vi "GenPointAttay.vi"(8 "error in":errorcluster, 11 "Option":T1={"X個數"=20, "Y個數"=10, "起始X"=0.0, "起始Y"=0.0, "位移X"=20.0, "位移Y"=20.0, "抖動range"=0.0}) -> (0 "error out":errorcluster, 3 "Output Points":cluster{"X":dbl, "Y":dbl}[](array[cluster]))   [LabVIEW 2015]
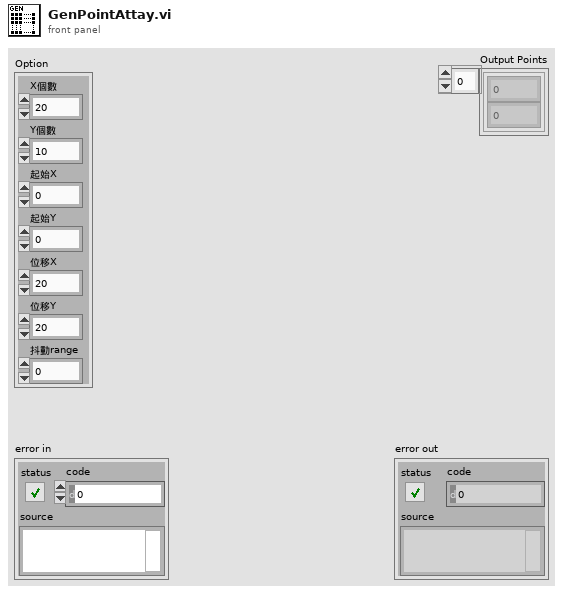
[diagram p1: front panel]
types:
  T1 = cluster{"X個數":i32, "Y個數":i32, "起始X":dbl, "起始Y":dbl, "位移X":dbl, "位移Y":dbl, "抖動range":dbl}
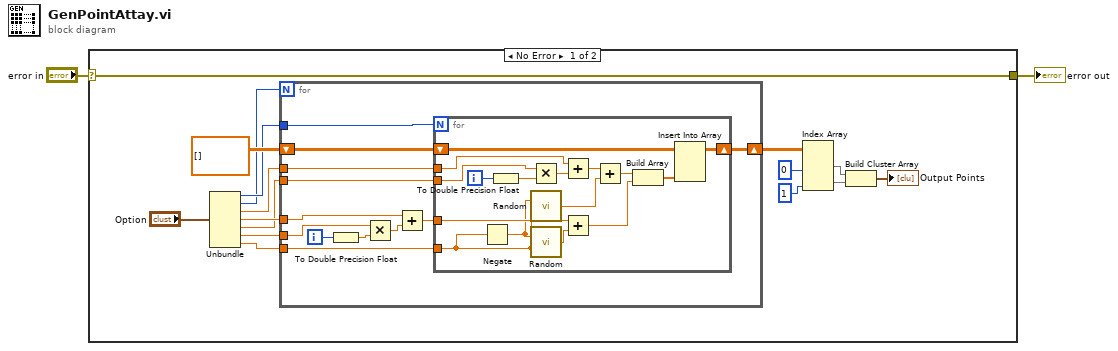
[diagram p0: block diagram]
diagram:
  n1 = case shown="No Error" "error in" {
    selector: "error in" -> [w3 w47]
    tunnel: [w3 w47] -> w1
    frame No Error {
      n2 = Unbundle("Option") -> ("X個數"=w10:i32, "Y個數"=w9:i32, "起始X"=w8:dbl, "起始Y"=w7:dbl, "位移X"=w6:dbl, "位移Y"=w5:dbl, "抖動range"=w4:dbl)
      n3 = for {
        N: w9 -> [_]
        shift-right: [w29] -> w13
        shift-left: dbl[][] [] -> [w30]
        tunnel: w8 -> [w26]
        tunnel: w7 -> [w25]
        tunnel: w6 -> [w24]
        tunnel: w5 -> [w23]
        tunnel: w4 -> [w22]
        tunnel: w10 -> [w21]
        i -> [w20]
        n4 = To Double Precision Float(number=w20) -> (double precision float=w19:dbl)
        n5 = Multiply(x=w23, y=w19) -> (x*y=w28:dbl)
        n6 = Add(x=w25, y=w28) -> (x+y=w27:dbl)
        n7 = for {
          N: w21 -> [_]
          shift-right: [w45] -> w29
          shift-left: w30 -> [w46]
          tunnel: w27 -> [w39]
          tunnel: w26 -> [w43]
          tunnel: w24 -> [w41]
          tunnel: w22 -> [w32]
          i -> [w34]
          n8 = Negate(x=w32) -> (-x=w31:dbl)
          n9 = To Double Precision Float(number=w34) -> (double precision float=w33:dbl)
          n10 = Multiply(x=w41, y=w33) -> (x*y=w42:dbl)
          n11 = call <userlib>:"Random.vi"("Min(0)"=w31, "Max"=w32) -> ("Random"=w35:dbl)  [unwired: 13 in]
          n12 = call <userlib>:"Random.vi"("Min(0)"=w31, "Max"=w32) -> ("Random"=w36:dbl)  [unwired: 13 in]
          n13 = Add(x=w43, y=w42) -> (x+y=w40:dbl)
          n14 = Add(x=w39, y=w36) -> (x+y=w38:dbl)
          n15 = Add(x=w40, y=w35) -> (x+y=w37:dbl)
          n16 = Build Array(w37, w38) -> (w44:dbl[])
          n17 = Insert Into Array(array=w46, new element=w44) -> (w45:dbl[][])  [unwired: 2 in]
        }
      }
      n18 = Index Array(array=w13, index (col) #1=0 ("disabled index (col)"), index (col) #2=1 ("index (col)")) -> (element #1=w14:dbl[], element #2=w15:dbl[])  [unwired: 2 in]
      n19 = Build Cluster Array(w14, w15) -> (→"Output Points":cluster{"Y":dbl, "Y":dbl}[])
    }
    frame Error {
    }
  }
  "error out" <- w1
